vi "MB Ethernet Call Wait on Query.vi"(9 "Timeout":i32=5000, 11 "Connection ID":refnum<k5>) -> ()   [LabVIEW 2020]
panel:
  # "VI Name: MB Ethernet Call Wait on Query.vi\nPurpose: Dynamically calls MB Ethernet Wait on Query.vi"
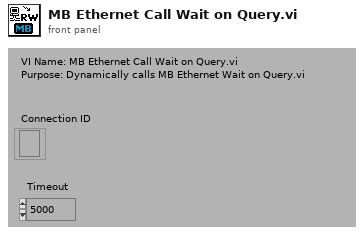
[diagram p1: front panel]
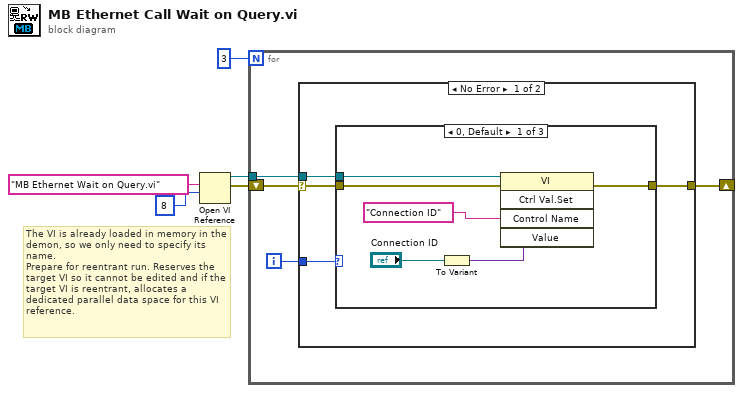
[diagram p0: block diagram]
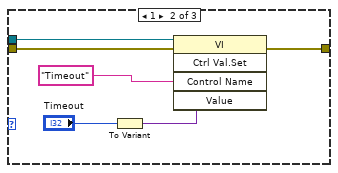
[diagram p2: hidden frame]
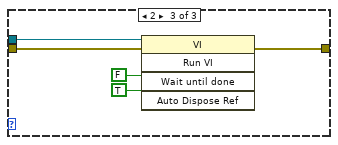
[diagram p3: hidden frame]
diagram:
  # "The VI is already loaded in memory in the demon, so we only need to specify its name.\nPrepare for reentrant run. Reserves the target VI so it cannot be edited and if the target VI is reentrant, allocates a dedicated parallel data space for this VI reference."
  n1 = Open VI Reference(vi path="MB Ethernet Wait on Query.vi", options=8) -> (vi reference=w5:refnum<vi>, error out=w4:errorcluster)  [unwired: 1 in, 3 out]
  n2 = for {
    N: 3 -> [_]
    tunnel: w5 -> [w9]
    shift-right: [w8] -> _
    shift-left: w4 -> [w7]
    i -> [w6]
    n3 = case shown="No Error" w7 {
      selector: w7 -> [w11 w31]
      tunnel: w9 -> [w13 _]
      tunnel: [w12 w31] -> w8
      tunnel: w6 -> [w10 _]
      frame No Error {
        n4 = case shown="0, Default" w10 {
          tunnel: w13 -> [w19 w25 w30]
          tunnel: w11 -> [w15 w22 w29]
          tunnel: [w14 w21 w28] -> w12
          frame 0, Default {
            n5 = To Variant(anything="Connection ID") -> (Variant=w16:variant)
            n6 = invoke class="VI" method="Ctrl Val.Set"(reference=w19, error in=w15, "Control Name"="Connection ID", "Value"=w16) -> (error out=w14:errorcluster)  [unwired: 1 in, 4 out]
          }
          frame 1 {
            n7 = To Variant(anything="Timeout") -> (Variant=w23:variant)
            n8 = invoke class="VI" method="Ctrl Val.Set"(reference=w25, error in=w22, "Control Name"="Timeout", "Value"=w23) -> (error out=w21:errorcluster)  [unwired: 1 in, 4 out]
          }
          frame 2 {
            n9 = invoke class="VI" method="Run VI"(reference=w30, error in=w29, "Wait until done"=FALSE, "Auto Dispose Ref"=TRUE) -> (error out=w28:errorcluster)  [unwired: 1 in, 4 out]
          }
        }
      }
      frame Error {
      }
    }
  }
